vi "Encoder Scaling VI.vi"(8 "Right Period (ticks/count)":i32=-5265301, 9 "Left Period (ticks/count)":i32=649830, 10 "Right Position (count)":i32, 11 "Left Position (count)":i32) -> (0 "Right Speed (inches/sec)":dbl=-0.16862120551132784, 1 "Left Speed (inches/sec)":dbl=1.3662671806472462, 2 "Right Position (inches)":dbl, 3 "Left Position (inches)":dbl)   [LabVIEW 2019]
uses:
  <vilib>/Analysis/3filter.llb/Filter Passband Type.ctl
  <vilib>/ptbypt/NI_PtbyPt.lvlib
  <vilib>/Analysis/NI_AALBase.lvlib
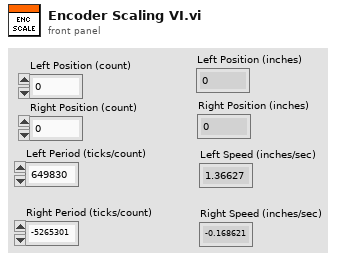
[diagram p1: front panel]
types:
  T1 = typedef "NI_AALBase.lvlib/Filter Passband Type.ctl" = enum32{"Lowpass", "Highpass", "Bandpass", "Bandstop"}
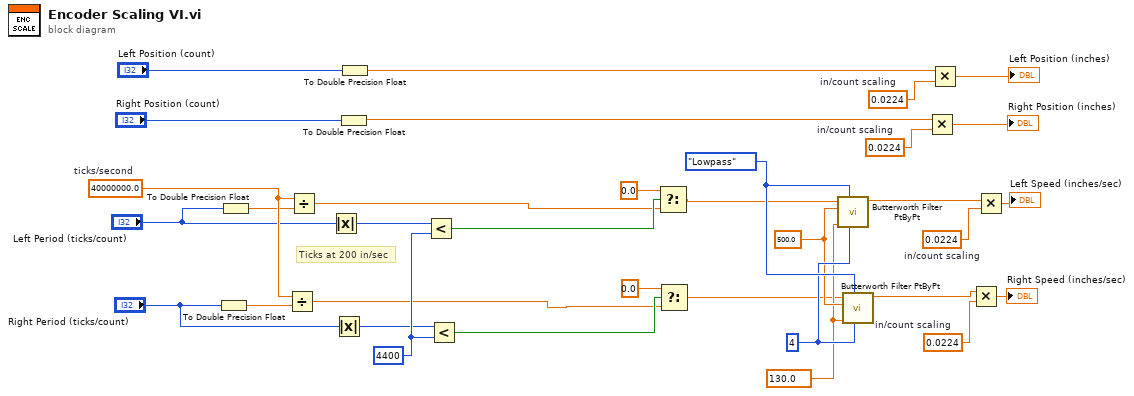
[diagram p0: block diagram]
diagram:
  w1 = 0.0224  # in/count scaling
  w5 = 0.0224  # in/count scaling
  w8 = 0.0224  # in/count scaling
  w11 = 0.0224  # in/count scaling
  w23 = 130.0 ("Sensor Cutoff Freq")
  w25 = 4 ("order")
  w26 = Filter_Passband_Type."Lowpass" ("filter type")
  w24 = 500.0 ("sampling freq: fs")
  w31 = 4400 ("y")
  w34 = 40000000.0  # ticks/second
  # "Ticks at 200 in/sec"
  n1 = To Double Precision Float(number="Right Period (ticks/count)") -> (double precision float=w15:dbl)
  n2 = To Double Precision Float(number="Left Period (ticks/count)") -> (double precision float=w18:dbl)
  n3 = Divide(x=w34, y=w15) -> (x/y=w13:dbl)
  n4 = Divide(x=w34, y=w18) -> (x/y=w14:dbl)
  n5 = Absolute Value(x="Left Period (ticks/count)") -> (abs(x)=w28:i32)
  n6 = Absolute Value(x="Right Period (ticks/count)") -> (abs(x)=w27:i32)
  n7 = To Double Precision Float(number="Right Position (count)") -> (double precision float=w7:dbl)
  n8 = To Double Precision Float(number="Left Position (count)") -> (double precision float=w12:dbl)
  n9 = Less?(x=w28, y=w31) -> (x < y?=w33:bool)
  n10 = Less?(x=w27, y=w31) -> (x < y?=w30:bool)
  n11 = Select(t=0.0 ("ticks/second"), s=w33, f=w14) -> (s? t:f=w22:dbl)
  n12 = Select(t=0.0 ("ticks/second"), s=w30, f=w13) -> (s? t:f=w21:dbl)
  n13 = call <vilib>:"Butterworth Filter PtByPt.vi"("order"=w25, "filter type"=w26, "low cutoff freq: fl"=w23, "sampling freq: fs"=w24, "x"=w22) -> ("Filtered x"=w6:dbl)  [unwired: 4 in, 1 out]
  n14 = call <vilib>:"Butterworth Filter PtByPt.vi"("order"=w25, "filter type"=w26, "low cutoff freq: fl"=w23, "sampling freq: fs"=w24, "x"=w21) -> ("Filtered x"=w2:dbl)  [unwired: 4 in, 1 out]
  n15 = Multiply(x=w7, y=w8) -> (x*y=→"Right Position (inches)":dbl)
  n16 = Multiply(x=w12, y=w11) -> (x*y=→"Left Position (inches)":dbl)
  n17 = Multiply(x=w2, y=w1) -> (x*y=→"Right Speed (inches/sec)":dbl)
  n18 = Multiply(x=w6, y=w5) -> (x*y=→"Left Speed (inches/sec)":dbl)
